vi "SPI Configure.vi"(7 "SPI Channel (0)":u8, 8 "Error In":errorcluster, 10 "SPI Configuration":T1={"Clock Frequency"=1000000, "Bit Order"=enum."LSb First", "SPI Mode"=enum."Mode 0"}, 11 "LINX Resource":T4) -> (0 "Error Out":errorcluster, 2 "Actual Clock Frequency":u32, 3 "LINX Resource":T4)   [LabVIEW 2014, in "LMH-LINX.lvlib"]
doc: "Configure the specified SPI channel. \n\nIf the LINX device has a single SPI master it is channel 0. If the LINX device has more than one SPI master the logical first SPI master is channel 0, the next is channel 1, etc.\n\n<b>Clock Frequency</b> specifies the desired SPI clock frequency. Since supported clock frequencies vary by device, the highest supported frequency that is less than or equal to the specified frequency is used. The actual frequency used is returned.\n<b>Bit Order</b> specifies the order that the bits are shifted out. LSb for least significant bit first, MSb for most significant bit first.\n<b>SPI Mode</b>specifies the SPI mode which set the clock phase and polarity. \n\nSPI Mode: Chose the SPI mode to determine the clock idle value and sampling edge as follows:\nMode 0 - Clock idle low; data sampled on rising edge.\nMode 1 - Clock idle low; data sampled on faling edge.\nMode 2 - Clock idle high; data sampled on faling edge.\nMode 3 - Clock idle high; data sampled on rising edge."
uses:
  <vilib>/MakerHub/LINX/LMH-LINX.lvlib
  <vilib>/MakerHub/LINX/Private/Type Defs/LINX Ref.ctl
  <vilib>/MakerHub/LINX/Private/Type Defs/Platform.ctl
  <vilib>/MakerHub/LINX/Private/Type Defs/Interface.ctl
  <vilib>/MakerHub/LINX/Private/Device/Type Defs/LINX Device Config.ctl
  <vilib>/MakerHub/LINX/Private/Device/Type Defs/TCP Config.ctl
  <vilib>/MakerHub/LINX/Private/Device/Type Defs/Channels.ctl
  <vilib>/MakerHub/LINX/Private/Type Defs/Peripherals/SPI/SPI Configuration.ctl
  <vilib>/MakerHub/LINX/Private/Type Defs/Peripherals/SPI/SPI Bit Order.ctl
  <vilib>/MakerHub/LINX/Private/Type Defs/Peripherals/SPI/SPI Mode.ctl
  <vilib>/MakerHub/LINX/Private/Type Defs/Peripheral.ctl
  <vilib>/MakerHub/LINX/Private/Utilties/Generate Error.vi
  <vilib>/MakerHub/LINX/Private/Device/Device.lvlib
  <vilib>/MakerHub/LINX/Private/Local IO/Local IO.lvlib
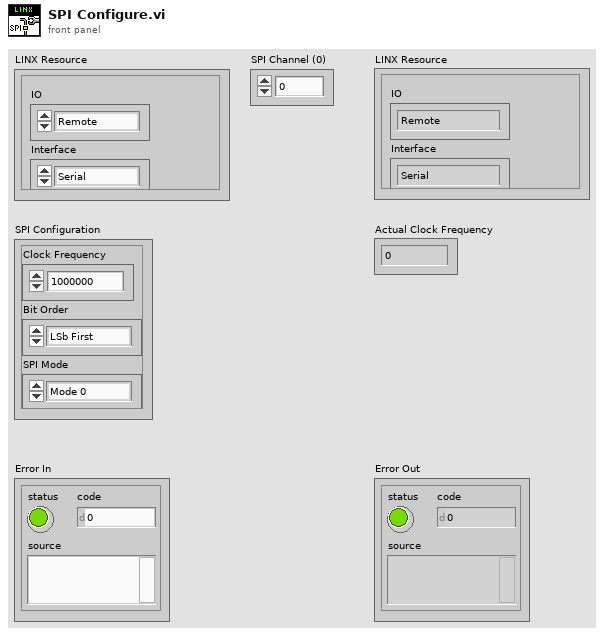
[diagram p1: front panel]
types:
  T1 = typedef "LMH-LINX.lvlib/SPI Configuration.ctl" = cluster{"Clock Frequency":u32, "Bit Order":T2, "SPI Mode":T3}
  T2 = typedef "LMH-LINX.lvlib/SPI Bit Order.ctl" = enum8{"LSb First", "MSb First"}
  T3 = typedef "LMH-LINX.lvlib/SPI Mode.ctl" = enum8{"Mode 0", "Mode 1", "Mode 2", "Mode 3"}
  T4 = typedef "LMH-LINX.lvlib/LINX Ref.ctl" = cluster{"IO":T5, "Interface":T6, "LINX Device Config":T7}
  T5 = typedef "LMH-LINX.lvlib/Platform.ctl" = enum16{"Remote", "Local"}
  T6 = typedef "LMH-LINX.lvlib/Interface.ctl" = enum16{"Serial", "TCP"}
  T7 = typedef "LMH-LINX.lvlib/Device.lvlib/LINX Device Config.ctl" = cluster{"Interface":T6, "COM Port":refnum<visa-resource-name>, "TCP Configuration":T8, "Device Family":u8, "Device ID":u8, "Device Name":string, "TCP Ref":refnum<k5>, "Channels":T9}
  T8 = typedef "LMH-LINX.lvlib/Device.lvlib/TCP Config.ctl" = cluster{"IP Address":string, "Port":u16}
  T9 = typedef "LMH-LINX.lvlib/Channels.ctl" = cluster{"DI":u8[], "DO":u8[], "AI":u8[], "AO":u8[], "PWM":u8[], "QE":u8[], "UART":u8[], "I2C 2":u8[], "SPI":u8[], "CAN":u8[], "Servo":u8[], "AI Ref (V)":dbl, "AI Resolution (Bits)":u8, "AO Ref (V)":dbl, "AO Resolution (Bits)":u8}
  T10 = typedef "LMH-LINX.lvlib/Peripheral.ctl" = enum8{"DI", "DO", "AI", "AO", "PWM", "QE", "UART", "I2C", "SPI", "CAN", "Servo"}
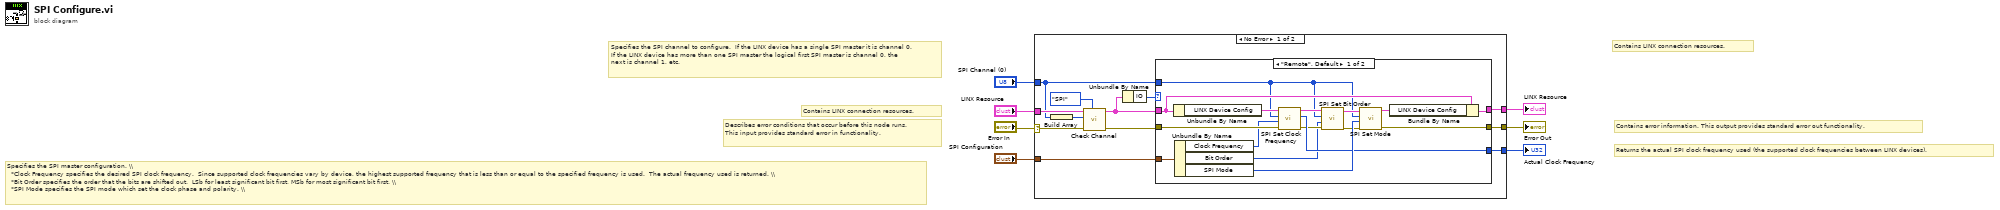
[diagram p0: block diagram]
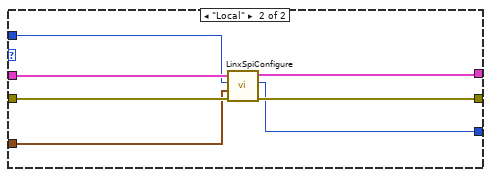
[diagram p2: hidden frame]
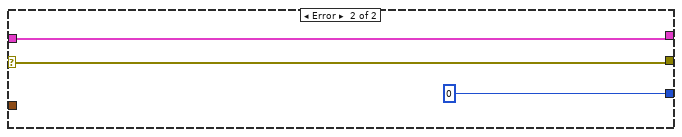
[diagram p3: hidden frame]
diagram:
  # "Returns the actual SPI clock frequency used (the supported clock frequencies between LINX devices)."
  # "Specifies the SPI channel to configure.  If the LINX device has a single SPI master it is channel 0.  If the LINX device has more than one SPI master the logical first SPI master is channel 0, the next is channel 1, etc."
  # "Specifies the SPI master configuration. \\\\\n  *Clock Frequency specifies the desired SPI clock frequency.  Since supported clock frequencies vary by device, the highest supported frequency that is less than or equal to the specified frequency is used.  The actual frequency used is returned. \\\\ \n  *Bit Order specifies the order that the bits are shifted out.  LSb for least significant bit first, MSb for most significant bit first. \\\\ \n  *SPI Mode specifies the SPI mode which set the clock phase and polarity. \\\\"
  # "Contains LINX connection resources."
  # "Contains error information. This output provides standard error out functionality."
  # "Contains LINX connection resources."
  # "Describes error conditions that occur before this node runs. This input provides standard error in functionality."
  n1 = case shown="No Error" "Error In" {
    selector: "Error In" -> [w9 w45]
    tunnel: [w18 w45] -> w7
    tunnel: [w17 w44] -> w6
    tunnel: "LINX Resource" -> [w16 w44]
    tunnel: "SPI Channel (0)" -> [w12 _]
    tunnel: "SPI Configuration" -> [w10 _]
    tunnel: [w8 u32 0 ("Actual Frequency")] -> w1
    frame No Error {
      n2 = Build Array(w12) -> (w13:u8[])
      n3 = call <vilib>:"Check Channel.vi"("Peripheral"=Peripheral."SPI", "Error In"=w9, "Channels"=w13, "LINX Resource"=w16) -> ("Error Out"=w14:errorcluster, "LINX Resource"=w15:T4)  [unwired: 5 in, 1 out]
      n4 = Unbundle By Name(w15) -> ("IO"=w19:T5)
      n5 = case shown="\"Remote\", Default" w19 {
        tunnel: w14 -> [w29 w41]
        tunnel: w15 -> [w35 w42]
        tunnel: [w31 w37] -> w18
        tunnel: [w34 w38] -> w17
        tunnel: w12 -> [w21 w39]
        tunnel: w10 -> [w33 w40]
        tunnel: [w26 w36] -> w8
        frame "Remote", Default {
          n6 = Unbundle By Name(w35) -> ("LINX Device Config"=w28:T7)
          n7 = Unbundle By Name(w33) -> ("Clock Frequency"=w27:u32, "Bit Order"=w20:T2, "SPI Mode"=w30:T3)
          n8 = call <vilib>:"SPI Set Clock Frequency.vi"("Error In"=w29, "Target Clock Frequency"=w27, "SPI Channel"=w21, "LINX Device Config"=w28) -> ("Error Out"=w23:errorcluster, "Actual Frequency"=w26:u32, "LINX Device Config"=w25:T7)  [unwired: 5 in]
          n9 = call <vilib>:"SPI Set Bit Order.vi"("Error In"=w23, "SPI Bit Order"=w20, "SPI Channel"=w21, "LINX Device Config"=w25) -> ("Error Out"=w22:errorcluster, "LINX Device Config"=w24:T7)  [unwired: 6 in]
          n10 = call <vilib>:"SPI Set Mode.vi"("Error In"=w22, "SPI Mode"=w30, "SPI Channel"=w21, "LINX Device Config"=w24) -> ("Error Out"=w31:errorcluster, "LINX Device Config"=w32:T7)  [unwired: 6 in]
          n11 = Bundle By Name(cluster=w35, "LINX Device Config"=w32) -> (w34:T4)
        }
        frame "Local" {
          n12 = call <vilib>:"LinxSpiConfigure.vi"("Error In"=w41, "SPI Configuration"=w40, "SPI Channel"=w39, "LINX Resource"=w42) -> ("Error Out"=w37:errorcluster, "actualSpeed"=w36:u32, "LINX Resource"=w38:T4)  [unwired: 5 in]
        }
      }
    }
    frame Error {
    }
  }
  "Error Out" <- w7
  "LINX Resource" <- w6
  "Actual Clock Frequency" <- w1
